vi "paint car.vi"(2 "Old Location":T1, 3 "New Location":T1, 5 "Map in":bool[][](array[boolean])) -> (0 "hit?":bool, 1 "Map out":bool[][](array[boolean]))   [LabVIEW 2020]
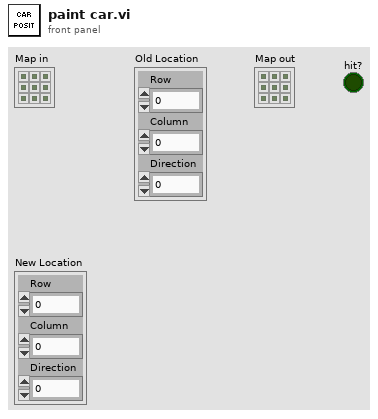
[diagram p1: front panel]
types:
  T1 = cluster{"Row":i32, "Column":i32, "Direction":i32}
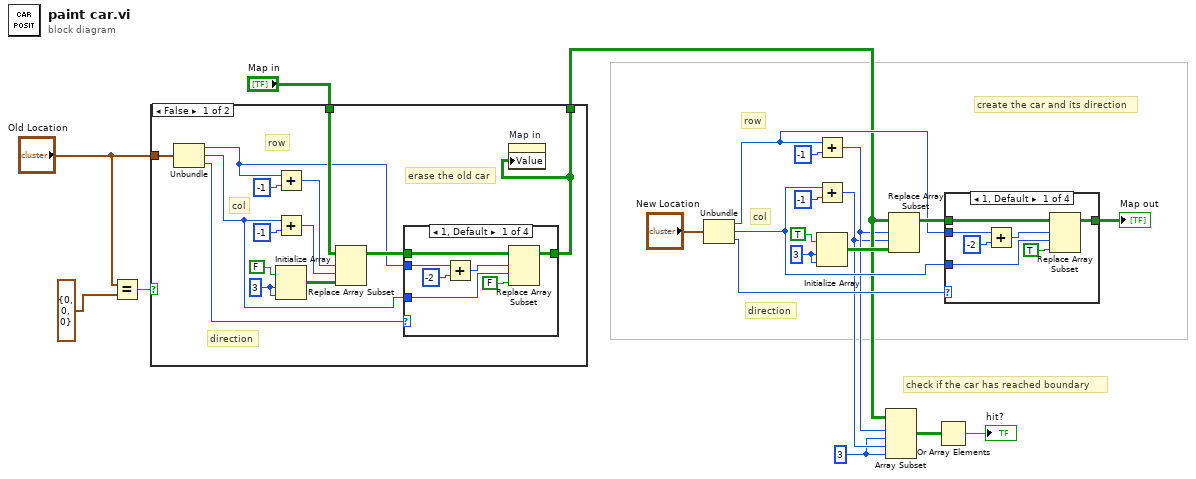
[diagram p0: block diagram]
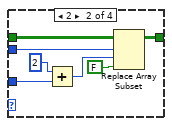
[diagram p2: hidden frame]
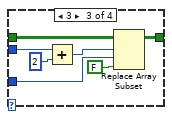
[diagram p3: hidden frame]
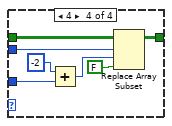
[diagram p4: hidden frame]
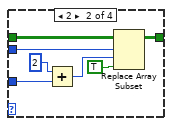
[diagram p6: hidden frame]
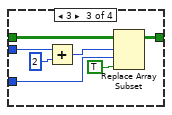
[diagram p7: hidden frame]
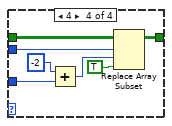
[diagram p8: hidden frame]
diagram:
  w3 = 3 ("length")
  w16 = 3 ("dimension size")
  # "check if the car has reached boundary"
  # "direction"
  # "col"
  # "row"
  # "create the car and its direction"
  n1 = Equal?(x="Old Location", y=T1 {"Row"=0, "Column"=0, "Direction"=0} ("Old Location")) -> (x = y?=w14:bool)
  n2 = case shown="False" w14 {
    tunnel: [w22 w64] -> w6
    tunnel: "Map in" -> [w27 w64]
    tunnel: "Old Location" -> [w26 _]
    frame False {
      w29 = 3 ("dimension size")
      # "direction"
      # "col"
      # "row"
      # "erase the old car"
      n3 = Unbundle(w26) -> ("Row"=w25:i32, "Column"=w24:i32, "Direction"=w23:i32)
      n4 = Add(x=w25, y=i64 -1) -> (x+y=w32:i64)
      n5 = Add(x=w24, y=i64 -1) -> (x+y=w34:i64)
      n6 = Initialize Array(FALSE, w29, w29) -> (w30:bool[][])
      n7 = Replace Array Subset(array=w27, new element=w30, index (row)=w32, index (col)=w34) -> (w31:bool[][])
      n8 = case shown="1, Default" w23 {
        tunnel: w31 -> [w42 w49 w56 w63]
        tunnel: w25 -> [w41 w45 w55 w59]
        tunnel: w24 -> [w40 w48 w54 w62]
        tunnel: [w36 w46 w50 w60] -> w22
        frame 1, Default {
          n9 = Add(x=w41, y=i64 -2) -> (x+y=w38:i64)
          n10 = Replace Array Subset(array=w42, new element=FALSE ("new element/subarray"), index (row)=w38, index (col)=w40) -> (w36:bool[][])
        }
        frame 2 {
          n11 = Add(x=i64 2, y=w48) -> (x+y=w44:i64)
          n12 = Replace Array Subset(array=w49, new element=FALSE ("new element/subarray"), index (row)=w45, index (col)=w44) -> (w46:bool[][])
        }
        frame 3 {
          n13 = Add(x=w55, y=i64 2) -> (x+y=w52:i64)
          n14 = Replace Array Subset(array=w56, new element=FALSE ("new element/subarray"), index (row)=w52, index (col)=w54) -> (w50:bool[][])
        }
        frame 4 {
          n15 = Add(x=i64 -2, y=w62) -> (x+y=w58:i64)
          n16 = Replace Array Subset(array=w63, new element=FALSE ("new element/subarray"), index (row)=w59, index (col)=w58) -> (w60:bool[][])
        }
      }
      n17 = property on="Map in" class="Arr (strict)"("Value"=w22) -> ()  [unwired: 2 in, 2 out]
    }
    frame True {
    }
  }
  n18 = Unbundle("New Location") -> ("Row"=w11:i32, "Column"=w10:i32, "Direction"=w9:i32)
  n19 = Add(x=w11, y=i64 -1) -> (x+y=w5:i64)
  n20 = Add(x=w10, y=i64 -1) -> (x+y=w4:i64)
  n21 = Initialize Array(TRUE, w16, w16) -> (w17:bool[][])
  n22 = Array Subset(array=w6, index (row)=w5, length (row)=w3, index (col)=w4, length (col)=w3) -> (w2:bool[][])
  n23 = Replace Array Subset(array=w6, new element=w17, index (row)=w5, index (col)=w4) -> (w18:bool[][])
  n24 = Or Array Elements(Boolean array=w2) -> (logical OR=→"hit?":bool)
  n25 = case shown="1, Default" w9 {
    tunnel: w18 -> [w71 w78 w85 w92]
    tunnel: w11 -> [w70 w74 w84 w88]
    tunnel: w10 -> [w69 w77 w83 w91]
    tunnel: [w65 w75 w79 w89] -> w19
    frame 1, Default {
      n26 = Add(x=w70, y=i64 -2) -> (x+y=w67:i64)
      n27 = Replace Array Subset(array=w71, new element=TRUE ("new element/subarray"), index (row)=w67, index (col)=w69) -> (w65:bool[][])
    }
    frame 2 {
      n28 = Add(x=i64 2, y=w77) -> (x+y=w73:i64)
      n29 = Replace Array Subset(array=w78, new element=TRUE ("new element/subarray"), index (row)=w74, index (col)=w73) -> (w75:bool[][])
    }
    frame 3 {
      n30 = Add(x=w84, y=i64 2) -> (x+y=w81:i64)
      n31 = Replace Array Subset(array=w85, new element=TRUE ("new element/subarray"), index (row)=w81, index (col)=w83) -> (w79:bool[][])
    }
    frame 4 {
      n32 = Add(x=i64 -2, y=w91) -> (x+y=w87:i64)
      n33 = Replace Array Subset(array=w92, new element=TRUE ("new element/subarray"), index (row)=w88, index (col)=w87) -> (w89:bool[][])
    }
  }
  "Map out" <- w19
